vi "Path Builder to Data Type.vi"(8 "error in (no error)":errorcluster, 11 "Path Builder":refnum<class "IPath Builder.lvclass">) -> (0 "error out":errorcluster, 3 "Boolean out":refnum<class "Path Builder.lvclass">)   [LabVIEW 2017, in "Custom Type Test Executive.lvlib" / "Path Builder.lvclass"]
uses:
  <vilib>/gpm_packages/@cs/test-executive/Source/Custom Type Test Executive/Path Builder Data Type/Path Builder.lvclass
  <vilib>/gpm_packages/@cs/test-executive/Source/Path Builder/IPath Builder/IPath Builder.lvclass
  <vilib>/gpm_packages/@cs/test-executive/Source/Custom Type Test Executive/Path Builder Data Type/Path Builder.lvclass/Path Builder.ctl
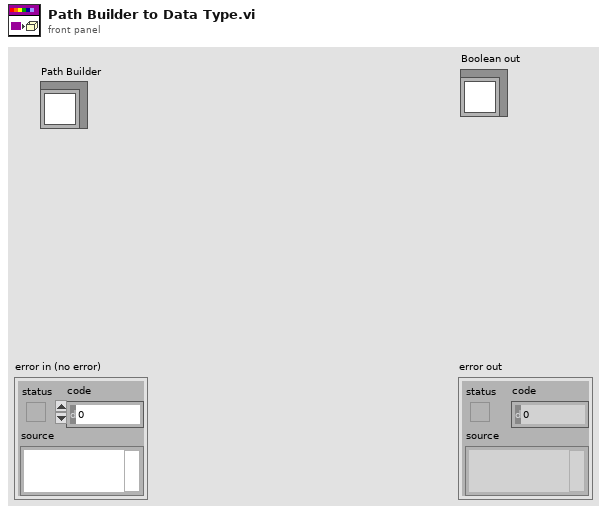
[diagram p1: front panel]
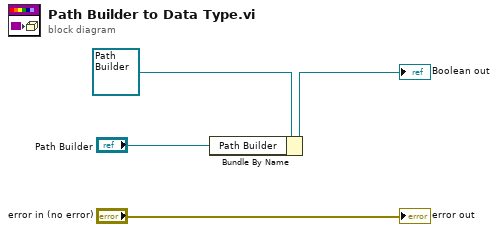
[diagram p0: block diagram]
diagram:
  n1 = Bundle By Name(cluster=refnum<class "Path Builder.lvclass"> refnum ("Boolean in"), "Path Builder"="Path Builder") -> (→"Boolean out":refnum<class "Path Builder.lvclass">)
  "error out" <- "error in (no error)"
